vi "CalculateMotorStartupTime.vi"(8 "error in (no error)":errorcluster, 9 "stop trigger level [RMS]":dbl format="%.2p", 10 "start trigger level [RMS]":dbl format="%.2p", 11 "waveform":waveform(dbl)) -> (0 "error out":errorcluster, 1 "startup start time":dbl, 3 "startup time":dbl)   [LabVIEW 2017, in "McsaAnalysisFunctions.lvlib"]
uses:
  <vilib>/addons/InsightCM/Utilities/Analysis/MCSA/McsaAnalysisFunctions.lvlib
  <vilib>/Waveform/WDTOps.llb/WDT Waveform Duration DBL.vi
  <vilib>/measure/mamon.llb/Trigger Detection for 1 Channel.vi
  <vilib>/measure/NI_MAPro.lvlib
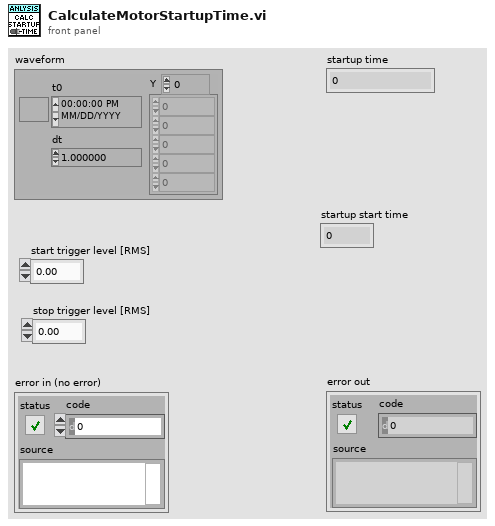
[diagram p1: front panel]
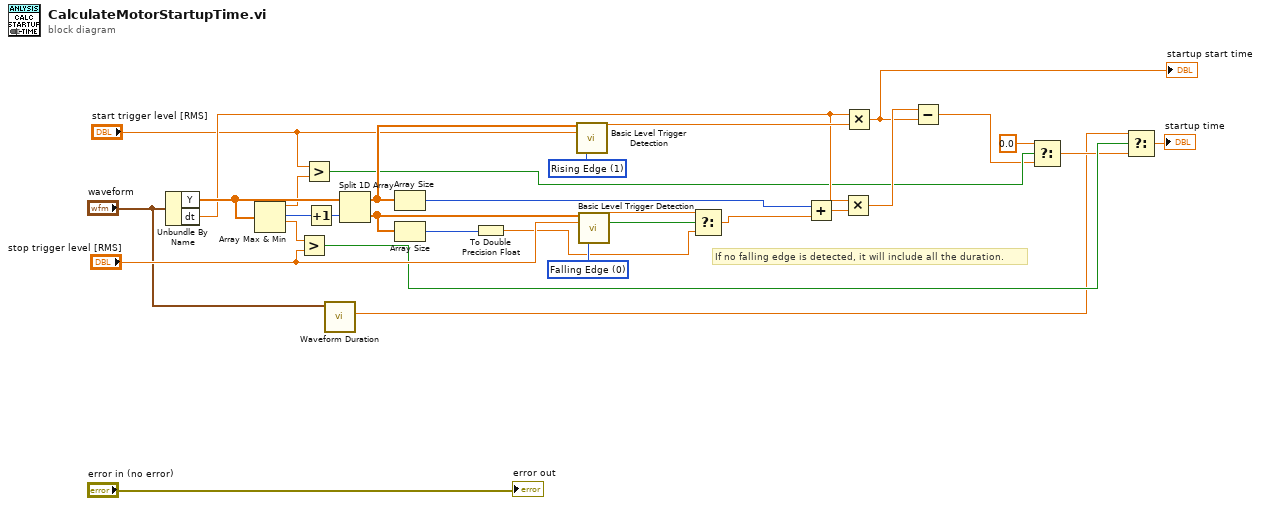
[diagram p0: block diagram]
diagram:
  w27 = u16 0 items=["Falling Edge", "Rising Edge"] ("trigger slope")
  w28 = u16 1 items=["Falling Edge", "Rising Edge"] ("trigger slope")
  # "If no falling edge is detected, it will include all the duration."
  n1 = Unbundle By Name("waveform") -> ("Y"=w18:dbl[], "dt"=w17:dbl)
  n2 = Array Max & Min(array=w18) -> (max value=w13:dbl, max index (indices)=w30:i32, min value=w20:dbl)  [unwired: 1 out]
  n3 = Greater?(x=w20, y="stop trigger level [RMS]") -> (0:w16:bool)
  n4 = Greater?(x="start trigger level [RMS]", y=w13) -> (0:w11:bool)
  n5 = Increment(x=w30) -> (x+1=w29:i32)
  n6 = call-poly <vilib>:"Waveform Duration.vi"("waveform in"="waveform") -> ("duration"=w7:dbl)  [unwired: 8 in, 2 out]
  n7 = Split 1D Array(array=w18, index=w29) -> (first subarray=w26:dbl[], second subarray=w6:dbl[])
  n8 = Array Size(array=w26) -> (size(s)=w25:i32)
  n9 = Array Size(array=w6) -> (size(s)=w1:i32)
  n10 = To Double Precision Float(number=w1) -> (double precision float=w2:dbl)
  n11 = call-poly <vilib>:"Basic Level Trigger Detection.vi"("signal in"=w26, "level"="start trigger level [RMS]", "trigger slope"=w28) -> ("trigger location"=w23:dbl)  [unwired: 10 in, 2 out]
  n12 = call-poly <vilib>:"Basic Level Trigger Detection.vi"("signal in"=w6, "level"="stop trigger level [RMS]", "trigger slope"=w27) -> ("trigger location"=w4:dbl, "trigger detected?"=w5:bool)  [unwired: 10 in, 1 out]
  n13 = Select(t=w4, s=w5, f=w2) -> (s? t:f=w3:dbl)
  n14 = Add(x=w25, y=w3) -> (x+y=w24:dbl)
  n15 = Multiply(x=w17, y=w24) -> (x*y=w22:dbl)
  n16 = Multiply(x=w17, y=w23) -> (x*y=w21:dbl)
  "startup start time" <- w21
  n17 = Subtract(x=w22, y=w21) -> (x-y=w8:dbl)
  n18 = Select(t=0.0, s=w11, f=w8) -> (s? t:f=w9:dbl)
  n19 = Select(t=w7, s=w16, f=w9) -> (s? t:f=→"startup time":dbl)
  "error out" <- "error in (no error)"
